vi "GUI_engineering.vi"(4 "error in (no error)":errorcluster) -> (0 "error out":errorcluster, 2 "Canceled?":bool)   [LabVIEW 2015]
doc: "An editor for the motor manager parameters. Use this GUI to change the global variables assoicated with each motor. This VI does not write the changes to an engineering file."
uses:
  GSCS Scripting/Utils/GSP_Wavelength_Global.vi
  Systems/Slit/GSP_SLIT_Global.vi
  Systems/Grating_Translation/GSP_GT_Global.vi
  Systems/Primary Filter/GSP_F1_Global.vi
  Systems/Secondary Filter/GSP_F2_Global.vi
  Systems/Cam_Focus/GSP_CF_Global.vi
panel:
  in  "Undo":bool
  in  "Apply and Exit":bool
  in  "Tab Control":T1(tab)
  in  "GS Degrees at Home":dbl=20.4 caption="Degrees at home" format="%.2f"
  in  "GS Ticks per Degree":dbl=10000.0 caption="Ticks/degree" format="%.2f"
  in  "C - G min":dbl
  in  "C - G max":dbl
  in  "Grating min":dbl
  in  "Grating max":dbl=44.0
  in  "Camera min":dbl=-1.0
  in  "Camera max":dbl=88.0
  in  "Degrees at home":dbl=15.0 format="%.4f"
  in  "Ticks/degree":dbl=28571.43 format="%.4f"
  in  "F1 Offset to 1st Pos SQUARE":i32 caption="Offset to 1st Pos SQR"
  in  "F1 Counts per Position SQUARE":dbl=6222.17 caption="Counts per Position SQR" format="%.2f"
  in  "F2 Offset to 1st Pos":i32 caption="Offset to 1st Pos"
  in  "F2 Counts per Position":dbl=6222.17 caption="Counts per Position" format="%.2f"
  in  "F1 Offset to 1st Pos":i32 caption="Offset to 1st Pos"
  in  "F1 Counts per Position":dbl=6222.17 caption="Counts per Position" format="%.2f"
  in  "Detent Position":i32
  in  "GT Offset to Clear Pos":i32=6580 caption="Offset to Clear Pos"
  in  "GT Offset between positions":i32=48715 caption="Offset Between Positions"
  in  "Offset to first Position":i32=175
  in  "Counts per Position":dbl=333.0 format="%.2f"
  in  "No Slit Position":i32=251743
  in  "Clear Position":i32=251743
  in  "Detent Position":i32=88865
  in  "Grab Position":i32=285543
  in  "Max Flex (deg)":dbl
  in  "B1 (microns)":dbl
  in  "Tilt (microns)":dbl
  in  "A2 (microns)":dbl
  in  "A1 (microns)":dbl
  # "Grating Stage"
  # "Interference (degrees)"
  # "Camera Stage"
  # "Primary Wheel (Square Holes)"
  # "Secondary Wheel"
  # "Primary Wheel (Round Holes)"
  # "Translation Stage"
  # "Translation Stage"
  # "Carousel"
  # "Camera offset = B1*(0.001/377.2)*\n\n(180/pi)*sin(rotator)"
  # "Camera stage"
  # "Left = -A1*cos(rotator)+(A2 + Tilt)*sin(rotator)+50\n\nRight = -A1*cos(rotator)+(A2 - Tilt)*sin(rotator)+50"
  # "Piezos"
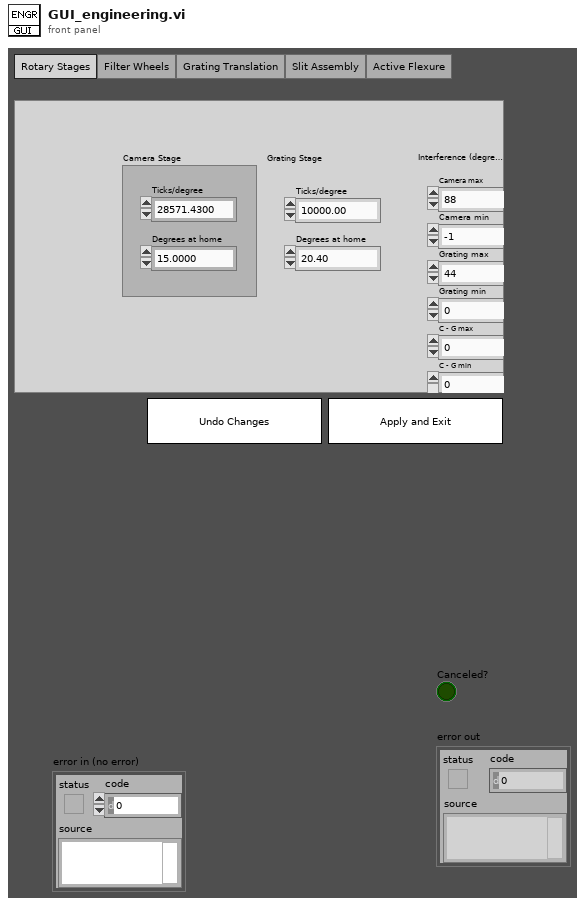
[diagram p1: front panel]
types:
  T1 = enum32{"Rotary Stages", "Filter Wheels", "Grating Translation", "Slit Assembly", "Active Flexure"}
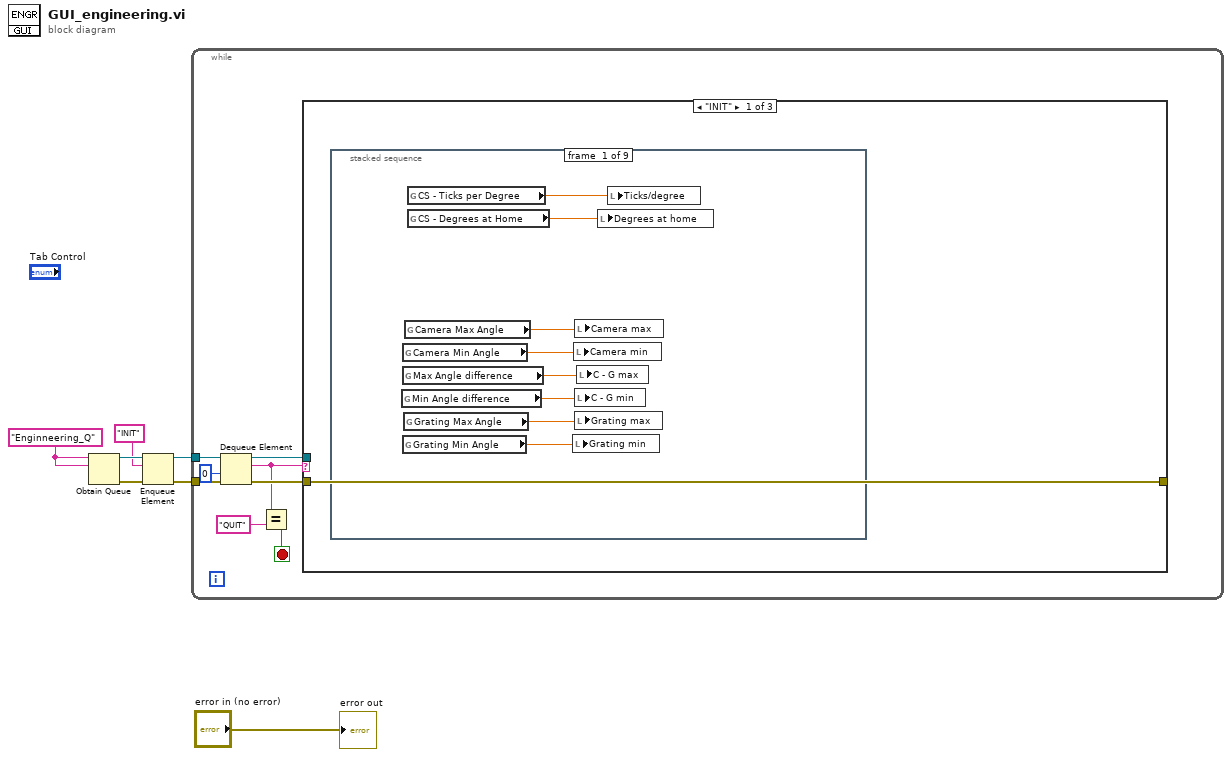
[diagram p0: block diagram]
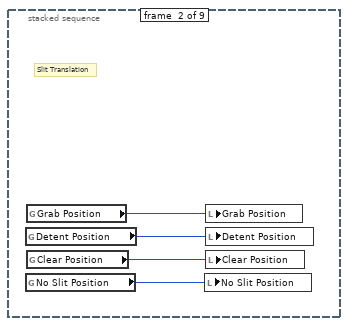
[diagram p2: hidden frame]
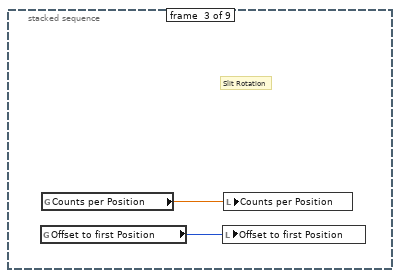
[diagram p3: hidden frame]
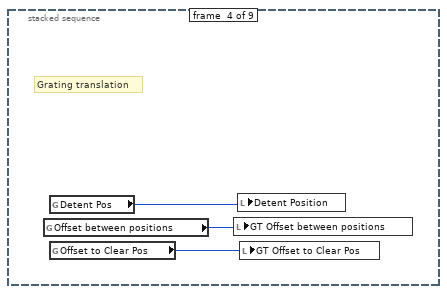
[diagram p4: hidden frame]
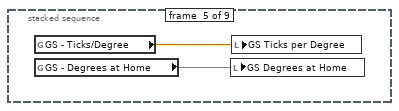
[diagram p5: hidden frame]
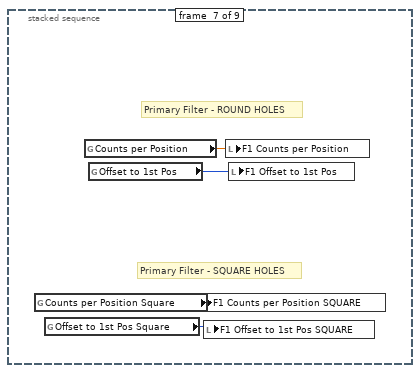
[diagram p7: hidden frame]
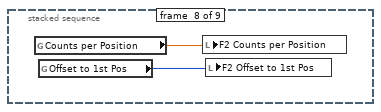
[diagram p8: hidden frame]
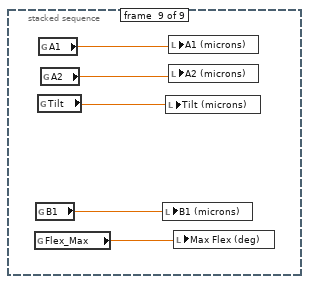
[diagram p9: hidden frame]
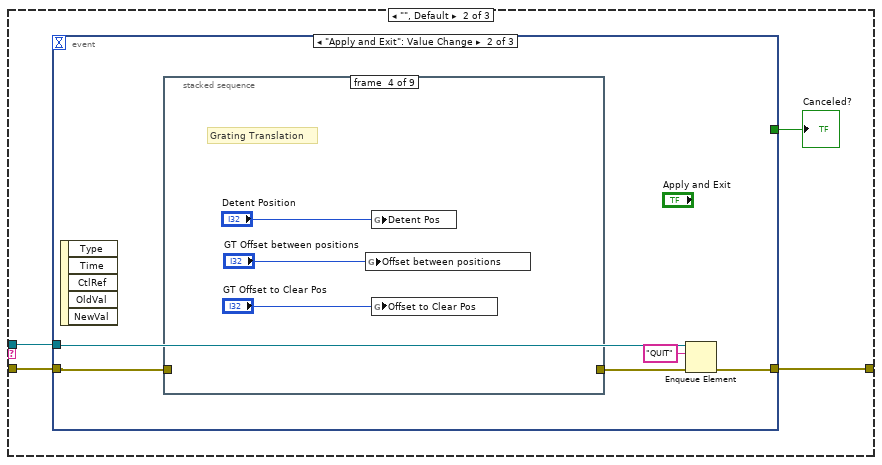
[diagram p10: hidden frame]
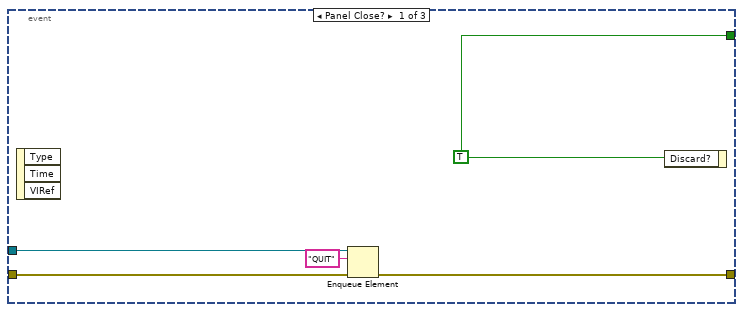
[diagram p11: hidden frame]
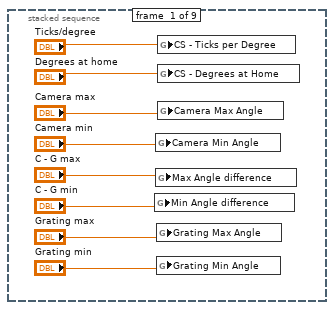
[diagram p12: hidden frame]
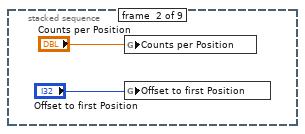
[diagram p13: hidden frame]
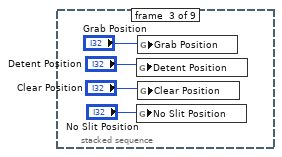
[diagram p14: hidden frame]
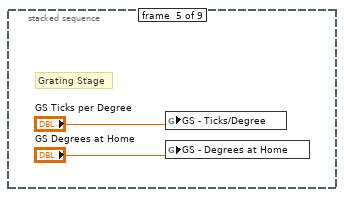
[diagram p15: hidden frame]
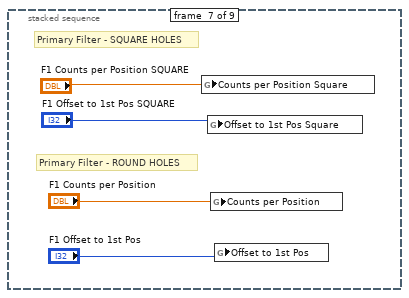
[diagram p17: hidden frame]
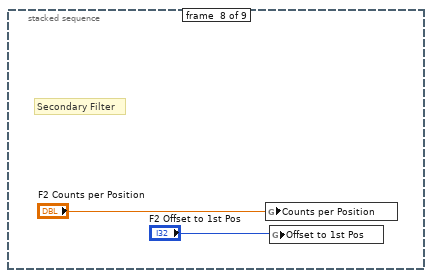
[diagram p18: hidden frame]
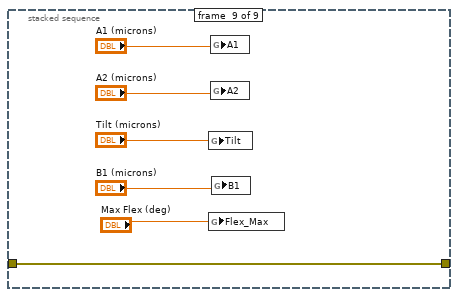
[diagram p19: hidden frame]
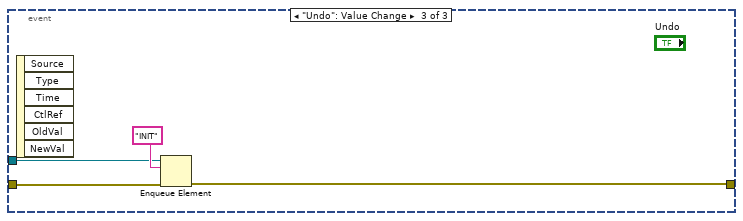
[diagram p20: hidden frame]
diagram:
  w3 = "Enginneering_Q"
  n1 = Obtain Queue(name (unnamed)=w3, element data type=w3) -> (queue out=w7:refnum<queue>, error out=w6:errorcluster)  [unwired: 3 in, 1 out]
  n2 = Enqueue Element(queue=w7, element="INIT", error in (no error)=w6) -> (queue out=w5:refnum<queue>, error out=w4:errorcluster)  [unwired: 1 in, 1 out]
  n3 = while {
    tunnel: w5 -> [w15]
    tunnel: w4 -> [w14]
    stop <- w9 stop-if-true
    n4 = Dequeue Element(queue=w15, timeout in ms (-1)=0, error in (no error)=w14) -> (queue out=w12:refnum<queue>, element=w11:string, error out=w13:errorcluster)  [unwired: 1 out]
    n5 = Equal?(x=w11, y="QUIT") -> (x = y?=w9:bool)
    n6 = case shown="\"INIT\"" w11 {
      tunnel: w13 -> [w16 w50 w96]
      tunnel: w12 -> [_ w49 _]
      tunnel: [w16 w48 w96] -> _
      frame "INIT" {
        n7 = stacked-sequence {
          frame #0 {
            n8 = global read "GSP_Wavelength_Global.vi" "Min Angle difference"() -> (w20:dbl)
            n9 = global read "GSP_Wavelength_Global.vi" "Camera Min Angle"() -> (w18:dbl)
            n10 = global read "GSP_Wavelength_Global.vi" "Max Angle difference"() -> (w19:dbl)
            n11 = global read "GSP_Wavelength_Global.vi" "Grating Min Angle"() -> (w22:dbl)
            n12 = global read "GSP_Wavelength_Global.vi" "Grating Max Angle"() -> (w21:dbl)
            n13 = global read "GSP_Wavelength_Global.vi" "Camera Max Angle"() -> (w17:dbl)
            n14 = global read "GSP_Wavelength_Global.vi" "CS - Ticks per Degree"() -> (w24:dbl)
            n15 = global read "GSP_Wavelength_Global.vi" "CS - Degrees at Home"() -> (w23:dbl)
            n16 = local write "Grating min"(w22) -> ()
            n17 = local write "Camera min"(w18) -> ()
            n18 = local write "Camera max"(w17) -> ()
            n19 = local write "C - G min"(w20) -> ()
            n20 = local write "Grating max"(w21) -> ()
            n21 = local write "C - G max"(w19) -> ()
            n22 = local write "Degrees at home"(w23) -> ()
            n23 = local write "Ticks/degree"(w24) -> ()
          }
          frame #1 {
            # "Slit Translation"
            n24 = global read "GSP_SLIT_Global.vi" "Detent Position"() -> (w27:i32)
            n25 = global read "GSP_SLIT_Global.vi" "No Slit Position"() -> (w25:i32)
            n26 = global read "GSP_SLIT_Global.vi" "Grab Position"() -> (w28:i32)
            n27 = global read "GSP_SLIT_Global.vi" "Clear Position"() -> (w26:i32)
            n28 = local write "No Slit Position"(w25) -> ()
            n29 = local write "Grab Position"(w28) -> ()
            n30 = local write "Detent Position"(w27) -> ()
            n31 = local write "Clear Position"(w26) -> ()
          }
          frame #2 {
            # "Slit Rotation"
            n32 = global read "GSP_SLIT_Global.vi" "Offset to first Position"() -> (w29:i32)
            n33 = global read "GSP_SLIT_Global.vi" "Counts per Position"() -> (w30:dbl)
            n34 = local write "Offset to first Position"(w29) -> ()
            n35 = local write "Counts per Position"(w30) -> ()
          }
          frame #3 {
            # "Grating translation"
            n36 = global read "GSP_GT_Global.vi" "Offset between positions"() -> (w32:i32)
            n37 = global read "GSP_GT_Global.vi" "Detent Pos"() -> (w31:i32)
            n38 = global read "GSP_GT_Global.vi" "Offset to Clear Pos"() -> (w33:i32)
            n39 = local write "GT Offset between positions"(w32) -> ()
            n40 = local write "Detent Position"(w31) -> ()
            n41 = local write "GT Offset to Clear Pos"(w33) -> ()
          }
          frame #4 {
            n42 = global read "GSP_Wavelength_Global.vi" "GS - Ticks/Degree"() -> (w35:dbl)
            n43 = global read "GSP_Wavelength_Global.vi" "GS - Degrees at Home"() -> (w34:dbl)
            n44 = local write "GS Degrees at Home"(w34) -> ()
            n45 = local write "GS Ticks per Degree"(w35) -> ()
          }
          frame #5 {
          }
          frame #6 {
            # "Primary Filter - SQUARE HOLES"
            # "Primary Filter - ROUND HOLES"
            n46 = global read "GSP_F1_Global.vi" "Counts per Position Square"() -> (w36:dbl)
            n47 = global read "GSP_F1_Global.vi" "Offset to 1st Pos Square"() -> (w37:i32)
            n48 = global read "GSP_F1_Global.vi" "Counts per Position"() -> (w39:dbl)
            n49 = global read "GSP_F1_Global.vi" "Offset to 1st Pos"() -> (w38:i32)
            n50 = local write "F1 Counts per Position SQUARE"(w36) -> ()
            n51 = local write "F1 Offset to 1st Pos SQUARE"(w37) -> ()
            n52 = local write "F1 Counts per Position"(w39) -> ()
            n53 = local write "F1 Offset to 1st Pos"(w38) -> ()
          }
          frame #7 {
            n54 = global read "GSP_F2_Global.vi" "Counts per Position"() -> (w40:dbl)
            n55 = global read "GSP_F2_Global.vi" "Offset to 1st Pos"() -> (w41:i32)
            n56 = local write "F2 Counts per Position"(w40) -> ()
            n57 = local write "F2 Offset to 1st Pos"(w41) -> ()
          }
          frame #8 {
            n58 = global read "GSP_Wavelength_Global.vi" "Flex_Max"() -> (w42:dbl)
            n59 = global read "GSP_Wavelength_Global.vi" "B1"() -> (w46:dbl)
            n60 = global read "GSP_CF_Global.vi" "Tilt"() -> (w43:dbl)
            n61 = global read "GSP_CF_Global.vi" "A1"() -> (w45:dbl)
            n62 = global read "GSP_CF_Global.vi" "A2"() -> (w44:dbl)
            n63 = local write "B1 (microns)"(w46) -> ()
            n64 = local write "Tilt (microns)"(w43) -> ()
            n65 = local write "A1 (microns)"(w45) -> ()
            n66 = local write "A2 (microns)"(w44) -> ()
            n67 = local write "Max Flex (deg)"(w42) -> ()
          }
        }
      }
      frame "", Default {
        n68 = event shown="[1] \"Apply and Exit\": Value Change" {
          selector: _ -> [_ _ _]
          dyn-events: _ -> [_ _ _]
          timeout: _ -> [_ _ _]
          tunnel: w50 -> [w55 w57 w93]
          tunnel: w49 -> [w54 w59 w94]
          tunnel: [w52 w58 w92] -> w48
          tunnel: [w51 _ _] -> w47
          event Panel Close? {
            w51 = TRUE
            n69 = event-data() -> ()  [unwired: 1 in, 3 out]
            n70 = Enqueue Element(queue=w54, element="QUIT", error in (no error)=w55) -> (error out=w52:errorcluster)  [unwired: 1 in, 2 out]
            n71 = event-data("Discard?"=w51) -> ()  [unwired: 1 in, 1 out]
          }
          event "Apply and Exit": Value Change {
            n72 = event-data() -> ()  [unwired: 1 in, 5 out]
            n73 = stacked-sequence {
              tunnel: w57 -> [_ _ _ _ _ _ _ _ w91]
              tunnel: [_ _ _ _ _ _ _ _ w91] -> w56
              frame #0 {
                n74 = global write "GSP_Wavelength_Global.vi" "Min Angle difference"("C - G min") -> ()
                n75 = global write "GSP_Wavelength_Global.vi" "Camera Min Angle"("Camera min") -> ()
                n76 = global write "GSP_Wavelength_Global.vi" "Max Angle difference"("C - G max") -> ()
                n77 = global write "GSP_Wavelength_Global.vi" "Grating Max Angle"("Grating max") -> ()
                n78 = global write "GSP_Wavelength_Global.vi" "Grating Min Angle"("Grating min") -> ()
                n79 = global write "GSP_Wavelength_Global.vi" "CS - Ticks per Degree"("Ticks/degree") -> ()
                n80 = global write "GSP_Wavelength_Global.vi" "CS - Degrees at Home"("Degrees at home") -> ()
                n81 = global write "GSP_Wavelength_Global.vi" "Camera Max Angle"("Camera max") -> ()
              }
              frame #1 {
                n82 = global write "GSP_SLIT_Global.vi" "Counts per Position"("Counts per Position") -> ()
                n83 = global write "GSP_SLIT_Global.vi" "Offset to first Position"("Offset to first Position") -> ()
              }
              frame #2 {
                n84 = global write "GSP_SLIT_Global.vi" "Detent Position"("Detent Position") -> ()
                n85 = global write "GSP_SLIT_Global.vi" "No Slit Position"("No Slit Position") -> ()
                n86 = global write "GSP_SLIT_Global.vi" "Grab Position"("Grab Position") -> ()
                n87 = global write "GSP_SLIT_Global.vi" "Clear Position"("Clear Position") -> ()
              }
              frame #3 {
                # "Grating Translation"
                n88 = global write "GSP_GT_Global.vi" "Offset between positions"("GT Offset between positions") -> ()
                n89 = global write "GSP_GT_Global.vi" "Detent Pos"("Detent Position") -> ()
                n90 = global write "GSP_GT_Global.vi" "Offset to Clear Pos"("GT Offset to Clear Pos") -> ()
              }
              frame #4 {
                # "Grating Stage"
                n91 = global write "GSP_Wavelength_Global.vi" "GS - Ticks/Degree"("GS Ticks per Degree") -> ()
                n92 = global write "GSP_Wavelength_Global.vi" "GS - Degrees at Home"("GS Degrees at Home") -> ()
              }
              frame #5 {
                # "Coll Focus"
              }
              frame #6 {
                # "Primary Filter - SQUARE HOLES"
                # "Primary Filter - ROUND HOLES"
                n93 = global write "GSP_F1_Global.vi" "Counts per Position Square"("F1 Counts per Position SQUARE") -> ()
                n94 = global write "GSP_F1_Global.vi" "Offset to 1st Pos Square"("F1 Offset to 1st Pos SQUARE") -> ()
                n95 = global write "GSP_F1_Global.vi" "Counts per Position"("F1 Counts per Position") -> ()
                n96 = global write "GSP_F1_Global.vi" "Offset to 1st Pos"("F1 Offset to 1st Pos") -> ()
              }
              frame #7 {
                # "Secondary Filter"
                n97 = global write "GSP_F2_Global.vi" "Counts per Position"("F2 Counts per Position") -> ()
                n98 = global write "GSP_F2_Global.vi" "Offset to 1st Pos"("F2 Offset to 1st Pos") -> ()
              }
              frame #8 {
                n99 = global write "GSP_CF_Global.vi" "Tilt"("Tilt (microns)") -> ()
                n100 = global write "GSP_Wavelength_Global.vi" "Flex_Max"("Max Flex (deg)") -> ()
                n101 = global write "GSP_CF_Global.vi" "A1"("A1 (microns)") -> ()
                n102 = global write "GSP_CF_Global.vi" "A2"("A2 (microns)") -> ()
                n103 = global write "GSP_Wavelength_Global.vi" "B1"("B1 (microns)") -> ()
              }
            }
            n104 = Enqueue Element(queue=w59, element="QUIT", error in (no error)=w56) -> (error out=w58:errorcluster)  [unwired: 1 in, 2 out]
          }
          event "Undo": Value Change {
            n105 = event-data() -> ()  [unwired: 1 in, 6 out]
            n106 = Enqueue Element(queue=w94, element="INIT", error in (no error)=w93) -> (error out=w92:errorcluster)  [unwired: 1 in, 2 out]
          }
        }
        "Canceled?" <- w47
      }
      frame "QUIT" {
      }
    }
  }
  "error out" <- "error in (no error)"
